vi "BRig_dataExp_DAB_flipLR_nTrial.vi"() -> (2 "output_DAB_flipLR_nTrial":i32)   [LabVIEW 2014]
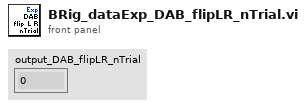
[diagram p1: front panel]
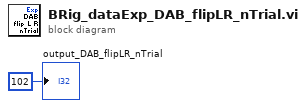
[diagram p0: block diagram]
diagram:
  "output_DAB_flipLR_nTrial" <- 102 ("output_iBlock")
